vi "read line from internal stream.vi"(8 "error in":errorcluster, 9 "max length":u64, 10 "delimiter":u8=10 format="%.0x", 11 "connection in":refnum<class "connection.lvclass">) -> (0 "error out":errorcluster, 3 "buffer":string)   [LabVIEW 2016, in "connection.lvclass"]
uses:
  connection.lvclass
  connection.lvclass/connection.ctl
  dllwrapper/library path.vi
  <vilib>/Utility/error.llb/Error Cluster From Error Code.vi
  dllwrapper/async tls dl.lvlib
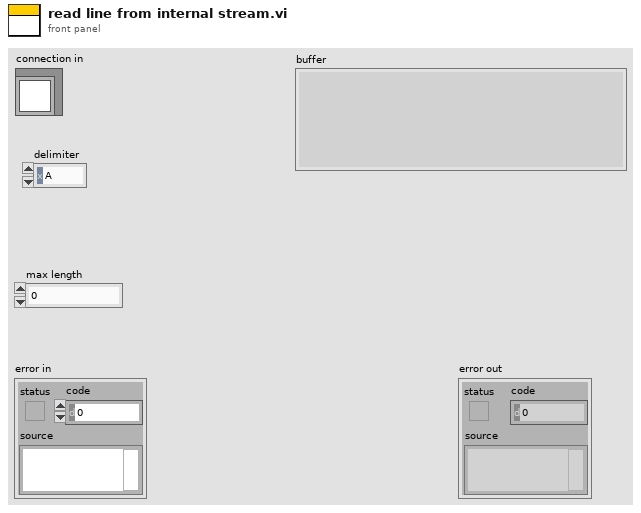
[diagram p1: front panel]
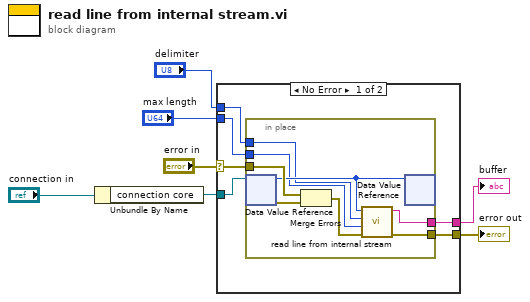
[diagram p0: block diagram]
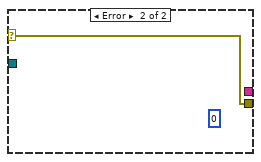
[diagram p2: hidden frame]
diagram:
  n1 = Unbundle By Name("connection in") -> ("connection core"=w6:refnum<data-value>)
  n2 = case shown="No Error" "error in" {
    selector: "error in" -> [w12 w22]
    tunnel: w6 -> [w13 _]
    tunnel: [w11 w22] -> w4
    tunnel: [w10 _] -> w3
    tunnel: "max length" -> [w9 _]
    tunnel: "delimiter" -> [w8 _]
    frame No Error {
      n3 = in-place {
        in-place-border: w12 -> [w21]
        in-place-border: [w18] -> w11
        in-place-border: [w16] -> w10
        in-place-border: w9 -> [w15]
        in-place-border: w8 -> [w14]
        n4 = in-place-dvr #1(w13) -> (w17:u64, w20:errorcluster)
        n5 = Merge Errors(w21, w20) -> (w19:errorcluster)
        n6 = call "read line from internal stream.vi"("error in"=w19, "max length"=w15, "delimiter"=w14, "socket"=w17) -> ("error out"=w18:errorcluster, "buffer"=w16:string)  [unwired: 6 in]
        n7 = in-place-dvr #1(w17) -> ()  [unwired: 2 out]
      }
    }
    frame Error {
      (unwired) u64 0 ("size")
    }
  }
  "error out" <- w4
  "buffer" <- w3
